vi "GetText.vi"(8 "error in":errorcluster, 11 "node in":refnum<class "VI modification collection.lvclass">) -> (0 "error out":errorcluster, 1 "additional text":string, 2 "text":string, 3 "node out":refnum<class "VI modification collection.lvclass">, 4 "glyph":string)   [LabVIEW 2013, in "VI modification collection.lvclass"]
doc: "Returns the text representation of the node used for the tree control."
uses:
  VI modification collection.lvclass
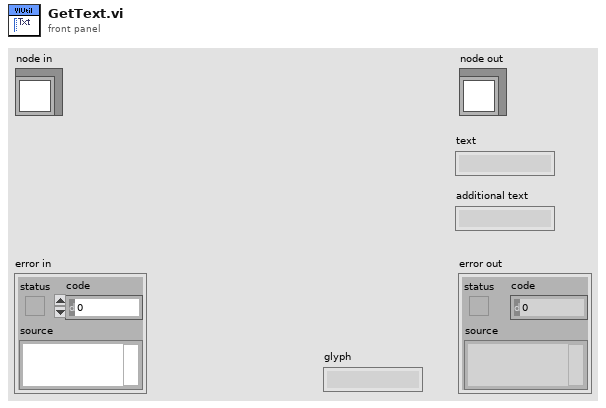
[diagram p1: front panel]
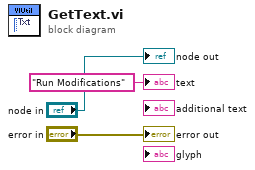
[diagram p0: block diagram]
diagram:
  "error out" <- "error in"
  "node out" <- "node in"
  "text" <- "Run Modifications" ("text")
